vi "construct_constant_array.vi"(1 "Low Mass Limit":i64, 2 "High Charge Limit":i16, 3 "High Mass Limit":i64, 4 "Low Velocity Count":i32, 5 "High Velocity Count":i32, 6 "Low Charge Limit":i16) -> (0 "Limits":T1={"High Charge Limit"=0, "Low Charge Limit"=0, "Time Out Limit"=0, "High Velocity Count"=0, "Low Velocity Count"=0, "Sampling Rate"=26666666.59375, "High Mass Limit"=0, "Low Mass Limit"=0})   [LabVIEW 2015]
uses:
  Limits.ctl
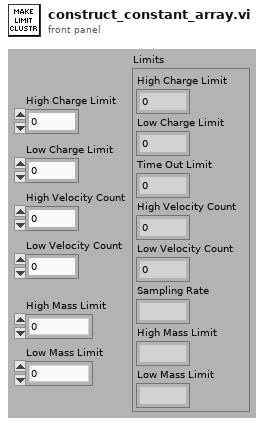
[diagram p1: front panel]
types:
  T1 = typedef "Limits.ctl" = cluster{"High Charge Limit":i16, "Low Charge Limit":i16, "Time Out Limit":i32, "High Velocity Count":i32, "Low Velocity Count":i32, "Sampling Rate":fxp<+,30,25>, "High Mass Limit":i64, "Low Mass Limit":i64}
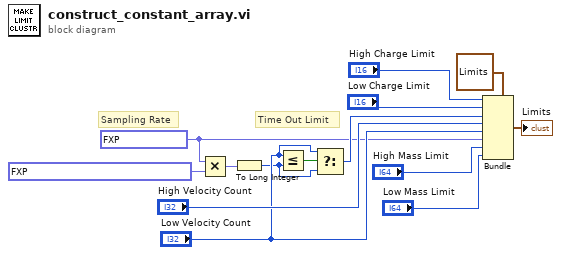
[diagram p0: block diagram]
diagram:
  w5 = fxp<+,30,25> 26666666.59375
  # "Sampling Rate"
  # "Time Out Limit"
  n1 = Multiply(x=w5, y=fxp<+,21,-8> 0.0034999996423721313) -> (x*y=w13:fxp<+,51,17>)
  n2 = To Long Integer(number=w13) -> (32bit integer=w7:i32)
  n3 = Less Or Equal?(x="Low Velocity Count", y=w7) -> (x <= y?=w9:bool)
  n4 = Select(t="Low Velocity Count", s=w9, f=w7) -> (s? t:f=w6:i32)
  n5 = Bundle(cluster=T1 {"High Charge Limit"=0, "Low Charge Limit"=0, "Time Out Limit"=0, "High Velocity Count"=0, "Low Velocity Count"=0, "Sampling Rate"=26666666.59375, "High Mass Limit"=0, "Low Mass Limit"=0} ("Limits"), "High Charge Limit"="High Charge Limit", "Low Charge Limit"="Low Charge Limit", "Time Out Limit"=w6, "High Velocity Count"="High Velocity Count", "Low Velocity Count"="Low Velocity Count", "Sampling Rate"=w5, "High Mass Limit"="High Mass Limit", "Low Mass Limit"="Low Mass Limit") -> (→"Limits":T1)
